vi "SM Initialize.vi"(8 "error in (no error)":errorcluster, 10 "Msg Queue":refnum<queue>, 11 "Message in":refnum<class "Message.lvclass">) -> (0 "error out":errorcluster, 3 "Message out":refnum<class "Message.lvclass">)   [LabVIEW 2020, in "OOP SM.lvlib"]
uses:
  OOP SM.lvlib
  Message/Message.lvclass
  Exe Msg/Exe Msg.lvclass
  E:/NI I Program/Actor Intr Demo/OOP SM/Message/Message.lvclass
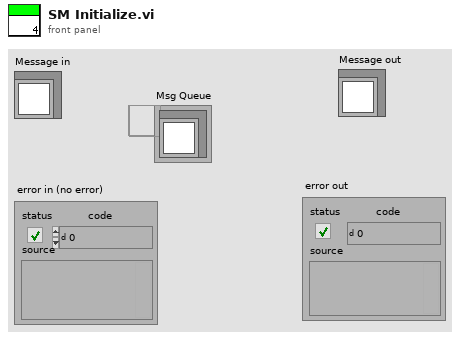
[diagram p1: front panel]
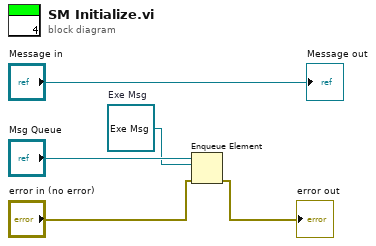
[diagram p0: block diagram]
diagram:
  w3 = refnum<class "Exe Msg.lvclass"> refnum  # Exe Msg
  n1 = Enqueue Element(queue="Msg Queue", element=w3, error in (no error)="error in (no error)") -> (error out=→"error out":errorcluster)  [unwired: 1 in, 2 out]
  "Message out" <- "Message in"
